vi "Reset.vi"(8 "error in (no error)":errorcluster, 11 "VISA resource name":refnum<visa-resource-name>) -> (0 "error out":errorcluster, 3 "VISA resource name out":refnum<visa-resource-name>)   [LabVIEW 2020, in "QuPMXdriver.lvlib"]
doc: "Resets the instrument .\nAll the slaves are opened (signal relays turned OFF and GND relays turned ON). Guard relays turned OFF. Local mode. Internal trigger. Status byte to default value."
uses:
  QuPMXdriver.lvlib
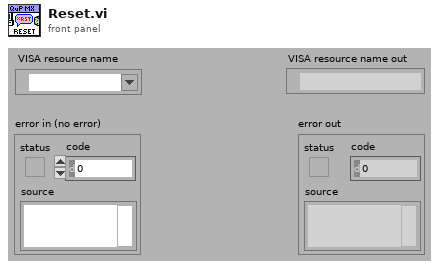
[diagram p1: front panel]
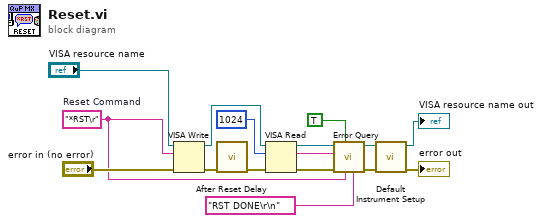
[diagram p0: block diagram]
diagram:
  w2 = "*RST\r"  # Reset Command
  n1 = VISA Write(VISA resource name="VISA resource name", write buffer=w2, error in (no error)="error in (no error)") -> (VISA resource name out=w10:refnum<visa-resource-name>, error out=w13:errorcluster)  [unwired: 1 out]
  n2 = call "After Reset Delay.vi"("error in"=w13) -> ("error out"=w11:errorcluster)  [unwired: 10 in]
  n3 = VISA Read(VISA resource name=w10, byte count=u32 1024, error in (no error)=w11) -> (VISA resource name out=w8:refnum<visa-resource-name>, read buffer=w3:string, error out=w9:errorcluster)  [unwired: 1 out]
  n4 = call "Error Query.vi"("Expected read buffer"="RST DONE\r\n" ("Correct answer"), "Last command"=w2, "Ignore empty sequence? (T)"=TRUE ("Ignore empty sequence?"), "error in (no error)"=w9, "Read buffer"=w3, "VISA resource name"=w8) -> ("error out"=w7:errorcluster, "VISA resource name out"=w4:refnum<visa-resource-name>)  [unwired: 4 in]
  n5 = call "Default Instrument Setup.vi"("error in (no error)"=w7, "VISA resource name"=w4) -> ("error out"=→"error out":errorcluster, "VISA resource name out"=→"VISA resource name out":refnum<visa-resource-name>)  [unwired: 8 in]
